vi "MSGR Send (Name).vi"(0 "Msg":string, 1 "MSGR Q name":T1, 5 "Parameters":string, 7 "Reply?":bool, 9 "ReplyQ":string, 11 "error in (no error)":errorcluster, 12 "timeout in ms (-1)":i32=-1) -> (8 "timed out?":bool, 15 "error out":errorcluster)   [LabVIEW 2018]
uses:
  MSGR Q Name TypeDef.ctl
  MSGR Q Data TypeDef.ctl
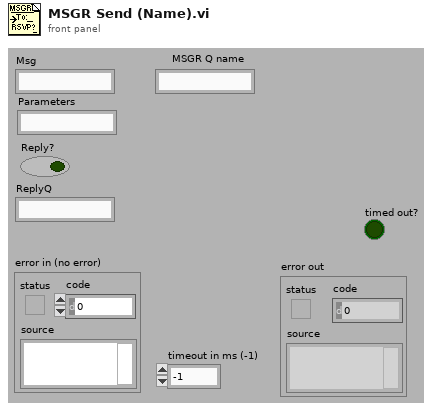
[diagram p1: front panel]
types:
  T1 = typedef "MSGR Q Name TypeDef.ctl" = string
  T2 = typedef "MSGR Q Data TypeDef.ctl" = cluster{"Msg":string, "Parameters":string, "Reply?":bool, "ReplyQ":string}
  T3 = typedef "MSGR Q Ref TypeDef.ctl" = refnum<queue>
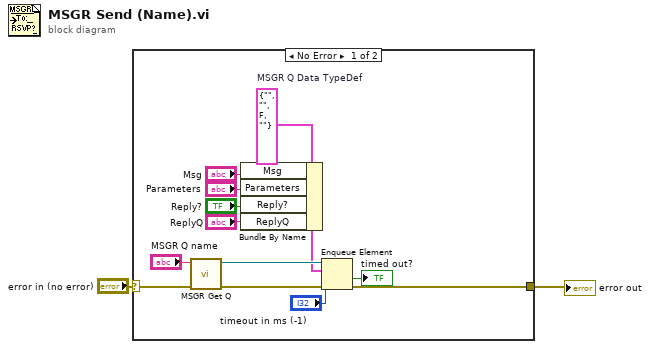
[diagram p0: block diagram]
diagram:
  n1 = case shown="No Error" "error in (no error)" {
    selector: "error in (no error)" -> [w15 w16]
    tunnel: [w7 w16] -> w2
    frame No Error {
      w4 = T2 {"Msg"="", "Parameters"="", "Reply?"=FALSE, "ReplyQ"=""}  # MSGR Q Data TypeDef
      n2 = call "MSGR Get Q.vi"("error in (no error)"=w15, "MSGR Q name"="MSGR Q name") -> ("error out"=w13:errorcluster, "MSGR Q"=w12:T3)  [unwired: 8 out]
      n3 = Bundle By Name(cluster=w4, "Msg"="Msg", "Parameters"="Parameters", "Reply?"="Reply?", "ReplyQ"="ReplyQ") -> (w11:T2)
      n4 = Enqueue Element(queue=w12, element=w11, timeout in ms (-1)="timeout in ms (-1)", error in (no error)=w13) -> (timed out?=→"timed out?":bool, error out=w7:errorcluster)  [unwired: 1 out]
    }
    frame Error {
    }
  }
  "error out" <- w2
